vi "Splash Screen.vi"(8 "error in":errorcluster) -> (0 "error out":errorcluster)   [LabVIEW 2019, in "Panther Dashboard.lvlib"]
uses:
  Panther Dashboard.lvlib
panel:
  out "Title and version":string
  # "info@pantherlab.com.mx"
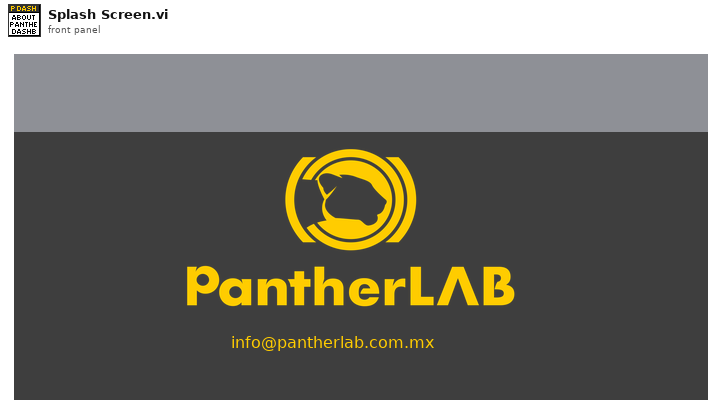
[diagram p1: front panel]
types:
  T1 = cluster{"Major":u16, "Minor":u16, "Fix":u16, "Build":u16}
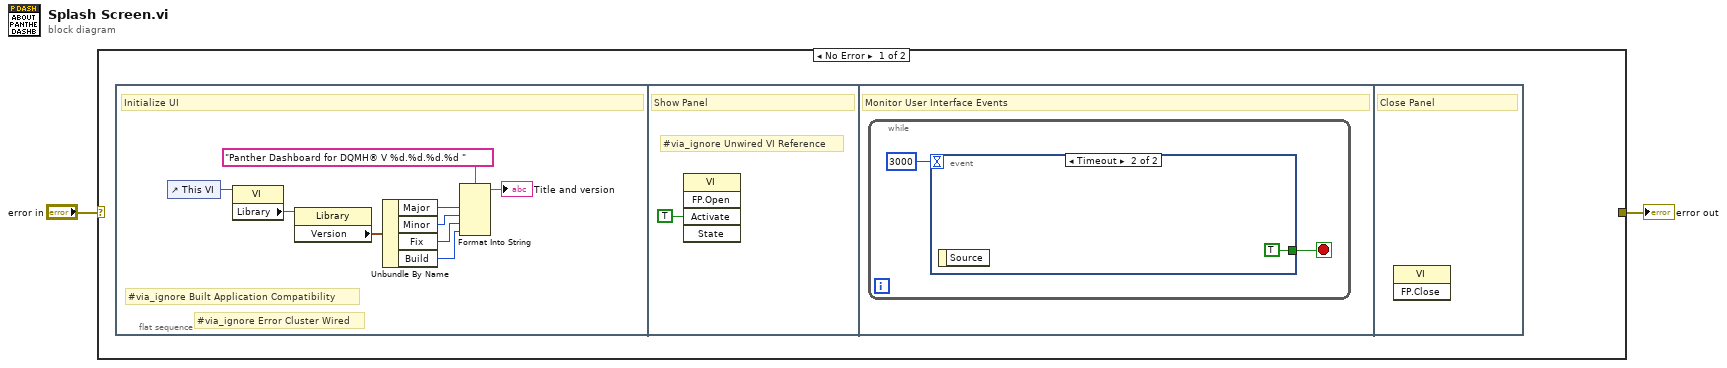
[diagram p0: block diagram]
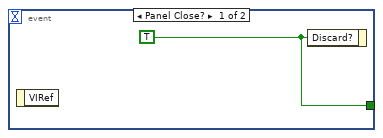
[diagram p2: hidden frame]
diagram:
  n1 = case shown="No Error" "error in" {
    selector: "error in" -> [_ w17]
    tunnel: [_ w17] -> w1
    frame No Error {
      n2 = flat-sequence {
        frame #0 {
          # "#via_ignore Built Application Compatibility"
          # "#via_ignore Error Cluster Wired"
          # "Initialize UI"
          n3 = control-ref of="This VI"() -> (w9:refnum<vi>)
          n4 = property class="VI"(reference=w9) -> ("Library"=w8:refnum<vi>)  [unwired: 1 in, 2 out]
          n5 = property class="Library"(reference=w8) -> ("Version"=w7:T1)  [unwired: 1 in, 2 out]
          n6 = Unbundle By Name(w7) -> ("Major"=w6:u16, "Minor"=w5:u16, "Fix"=w4:u16, "Build"=w3:u16)
          n7 = Format Into String(format string="Panther Dashboard for DQMH® V %d.%d.%d.%d " ("String"), w6, w5, w4, w3) -> (resulting string=→"Title and version":string)  [unwired: 2 in, 1 out]
        }
        frame #1 {
          # "#via_ignore Unwired VI Reference"
          # "Show Panel"
          n8 = invoke class="VI" method="FP.Open"("Activate"=TRUE ("Activate?")) -> ()  [unwired: 4 in, 5 out]
        }
        frame #2 {
          # "Monitor User Interface Events"
          n9 = while {
            stop <- w14 stop-if-true
            n10 = event shown="[1] Timeout" {
              selector: _ -> [_ _]
              dyn-events: _ -> [_ _]
              timeout: 3000 -> [_ _]
              tunnel: [w15 TRUE ("About DQMH")] -> w14
              event Panel Close? {
                w15 = TRUE ("Discard?")
                n11 = event-data() -> ()  [unwired: 1 in, 1 out]
                n12 = event-data("Discard?"=w15) -> ()  [unwired: 1 in, 1 out]
              }
              event Timeout {
                n13 = event-data() -> ()  [unwired: 1 in, 1 out]
              }
            }
          }
        }
        frame #3 {
          # "Close Panel"
          n14 = invoke class="VI" method="FP.Close"() -> ()  [unwired: 3 in, 3 out]
        }
      }
    }
    frame Error {
    }
  }
  "error out" <- w1
